vi "Teleop.vi"(10 "Match Info":T1={"Autonomous Elapsed Seconds"=0.0, "TeleOp Elapsed Seconds"=0.0, "Disabled Elapsed Seconds"=0.0, "Visited Autonomous"=FALSE, "Visited TeleOp"=FALSE, "Visited Disabled"=FALSE, "Autonomous Settings"={"Autonomous Style"=enum."Independent", "VI Refnum"=refnum}}, 11 "Call Context":T2) -> ()   [LabVIEW 2012]
doc: "This VI is called for each TeleOp packet received from the DS where the robot is not disabled. It is often used to read from the joysticks and update I/O or to update setpoints for timed control loops. It should complete and return within 20 milliseconds or it may miss DS packets."
uses:
  <vilib>/Rock Robotics/WPI/DriverStation/WPI_DriverStationDerivedRobotMode.ctl
  <vilib>/Rock Robotics/WPI/DriverStation/WPI_DriverStationMatch Info.ctl
  <vilib>/Rock Robotics/WPI/Relay/WPI_RelayValue.ctl
  Robot Global Data.vi
  <vilib>/Rock Robotics/WPI/Joystick/WPI_JoystickGetSetRefNum.vi
panel:
  in  "Numeric":dbl=0.87
  in  "Ext Const":dbl=0.5
  in  "Dep Const":dbl=1.0
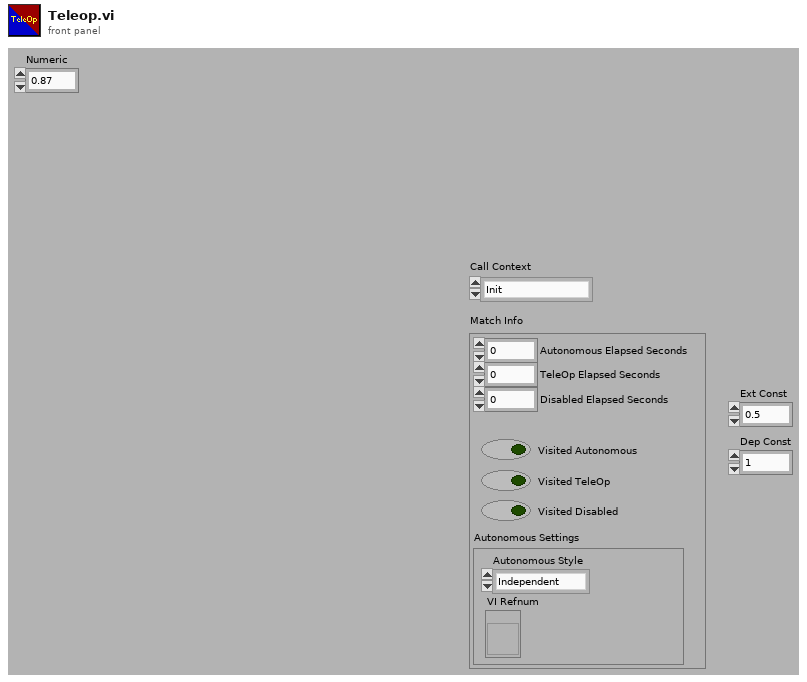
[diagram p1: front panel]
types:
  T1 = typedef "WPI_DriverStationMatch Info.ctl" = cluster{"Autonomous Elapsed Seconds":dbl, "TeleOp Elapsed Seconds":dbl, "Disabled Elapsed Seconds":dbl, "Visited Autonomous":bool, "Visited TeleOp":bool, "Visited Disabled":bool, "Autonomous Settings":cluster{"Autonomous Style":enum16{"Iterative", "Independent"}, "VI Refnum":refnum<vi>}}
  T2 = typedef "WPI_DriverStationDerivedRobotMode.ctl" = enum16{"Init", "Execute", "Stop"}
  T3 = typedef "WPI_RelayValue.ctl" = enum16{"Off", "On", "Forward", "Reverse"}
  T4 = cluster{"Driver Station Digital Input (1-8)[0]":bool, "Driver Station Digital Input (1-8)[1]":bool, "Driver Station Digital Input (1-8)[2]":bool, "Driver Station Digital Input (1-8)[3]":bool, "Driver Station Digital Input (1-8)[4]":bool, "Driver Station Digital Input (1-8)[5]":bool, "Driver Station Digital Input (1-8)[6]":bool, "Driver Station Digital Input (1-8)[7]":bool, "Driver Station Digital Input (1-8)[8]":bool}
  T5 = typedef "WPI_DigitalInputDevRef.ctl" = cluster{"DevStatus":errorcluster, "DIO Channel":T6, "Digital Module":T7}
  T6 = typedef "FPGA_DIOChannel.ctl" = enum8{"DIO 1", "DIO 2", "DIO 3", "DIO 4", "DIO 5", "DIO 6", "DIO 7", "DIO 8", "DIO 9", "DIO 10", "DIO 11", "DIO 12", "DIO 13", "DIO 14", "Invalid"}
  T7 = typedef "FPGA_TypedefDigitalModule.ctl" = enum16{"Digital Module 1", "Digital Module 2"}
  T8 = cluster{"Right Servo High":dbl, "Right Servo Mid":dbl, "Right Servo Low":dbl, "Left Servo High":dbl, "Left Servo Mid":dbl, "Left Servo Low":dbl}
  T9 = typedef "WPI_JoystickDevRef.ctl" = cluster{"Device":T10}
  T10 = typedef "WPI_JoystickDeviceEnum.ctl" = enum16{"USB 1", "USB 2", "USB 3", "USB 4", "Kinect 1", "Kinect 2"}
  T11 = cluster{"axis 1 (x)":dbl, "axis 2 (y)":dbl, "axis 3 (throttle)":dbl, "axis 4":dbl, "axis 5":dbl, "axis 6":dbl}
  T12 = typedef "WPI_RelayDevRef.ctl" = cluster{"DevStatus":errorcluster, "Relay Channel":T13, "Digital Module":T7, "Relay Direction":T14}
  T13 = typedef "FPGA_DIORelayChannel.ctl" = enum8{"Relay 1", "Relay 2", "Relay 3", "Relay 4", "Relay 5", "Relay 6", "Relay 7", "Relay 8", "Invalid"}
  T14 = typedef "WPI_RelayDirection.ctl" = enum16{"Both directions", "Forward only", "Reverse only"}
  T15 = typedef "WPI_ServoDeviceRef.ctl" = cluster{"DeviceStatus":errorcluster, "Digital Module":T7, "PWM Channel":T16, "DeadBand":T17}
  T16 = typedef "FPGA_DIOPWMChannel.ctl" = enum8{"PWM 1", "PWM 2", "PWM 3", "PWM 4", "PWM 5", "PWM 6", "PWM 7", "PWM 8", "PWM 9", "PWM 10", "Invalid"}
  T17 = typedef "WPI_PWMDeadband.ctl" = cluster{"Name":string, "maxPositivePwm":i32, "minPositivePwm":i32, "centerPwm":i32, "maxNegativePwm":i32, "minNegativePwm":i32, "angularRange":u16}
  T18 = typedef "WPI_MotorControlDeviceRef.ctl" = cluster{"DeviceStatus":errorcluster, "Type":enum16{"PWM", "CAN"}, "PWM":cluster{"Digital Module":T7, "PWM Channel":T16, "DeadBand":T17}, "CAN":cluster{"Device Number":u8, "Control Mode":T19, "Semaphore":T20, "Max Vout":dbl}, "Invert":bool, "TransformRef":T21, "InvTransformRef":T21}
  T19 = typedef "WPI_CANJaguar_ControlMode.ctl" = enum8{"Percent VBus", "Current", "Speed", "Position", "Voltage"}
  T20 = typedef "Semaphore RefNum" = refnum<k1>
  T21 = typedef "WPI_PWMTransform_ConPane.ctl" = refnum<vi>
  T22 = typedef "WPI_JoystickButtonState.ctl" = cluster{"Button 1":bool, "Button 2":bool, "Button 3":bool, "Button 4":bool, "Button 5":bool, "Button 6":bool, "Button 7":bool, "Button 8":bool, "Button 9":bool, "Button 10":bool, "Button 11":bool, "Button 12":bool}
  T23 = cluster{"FlipperLeftUp":dbl, "FlipperLeftDown":dbl, "FlipperRightUp":dbl, "FlipperRightDown":dbl, "KickerLeftBack":dbl, "KickerLeftForward":dbl, "KickerRightBack":dbl, "KickerRightForward":dbl}
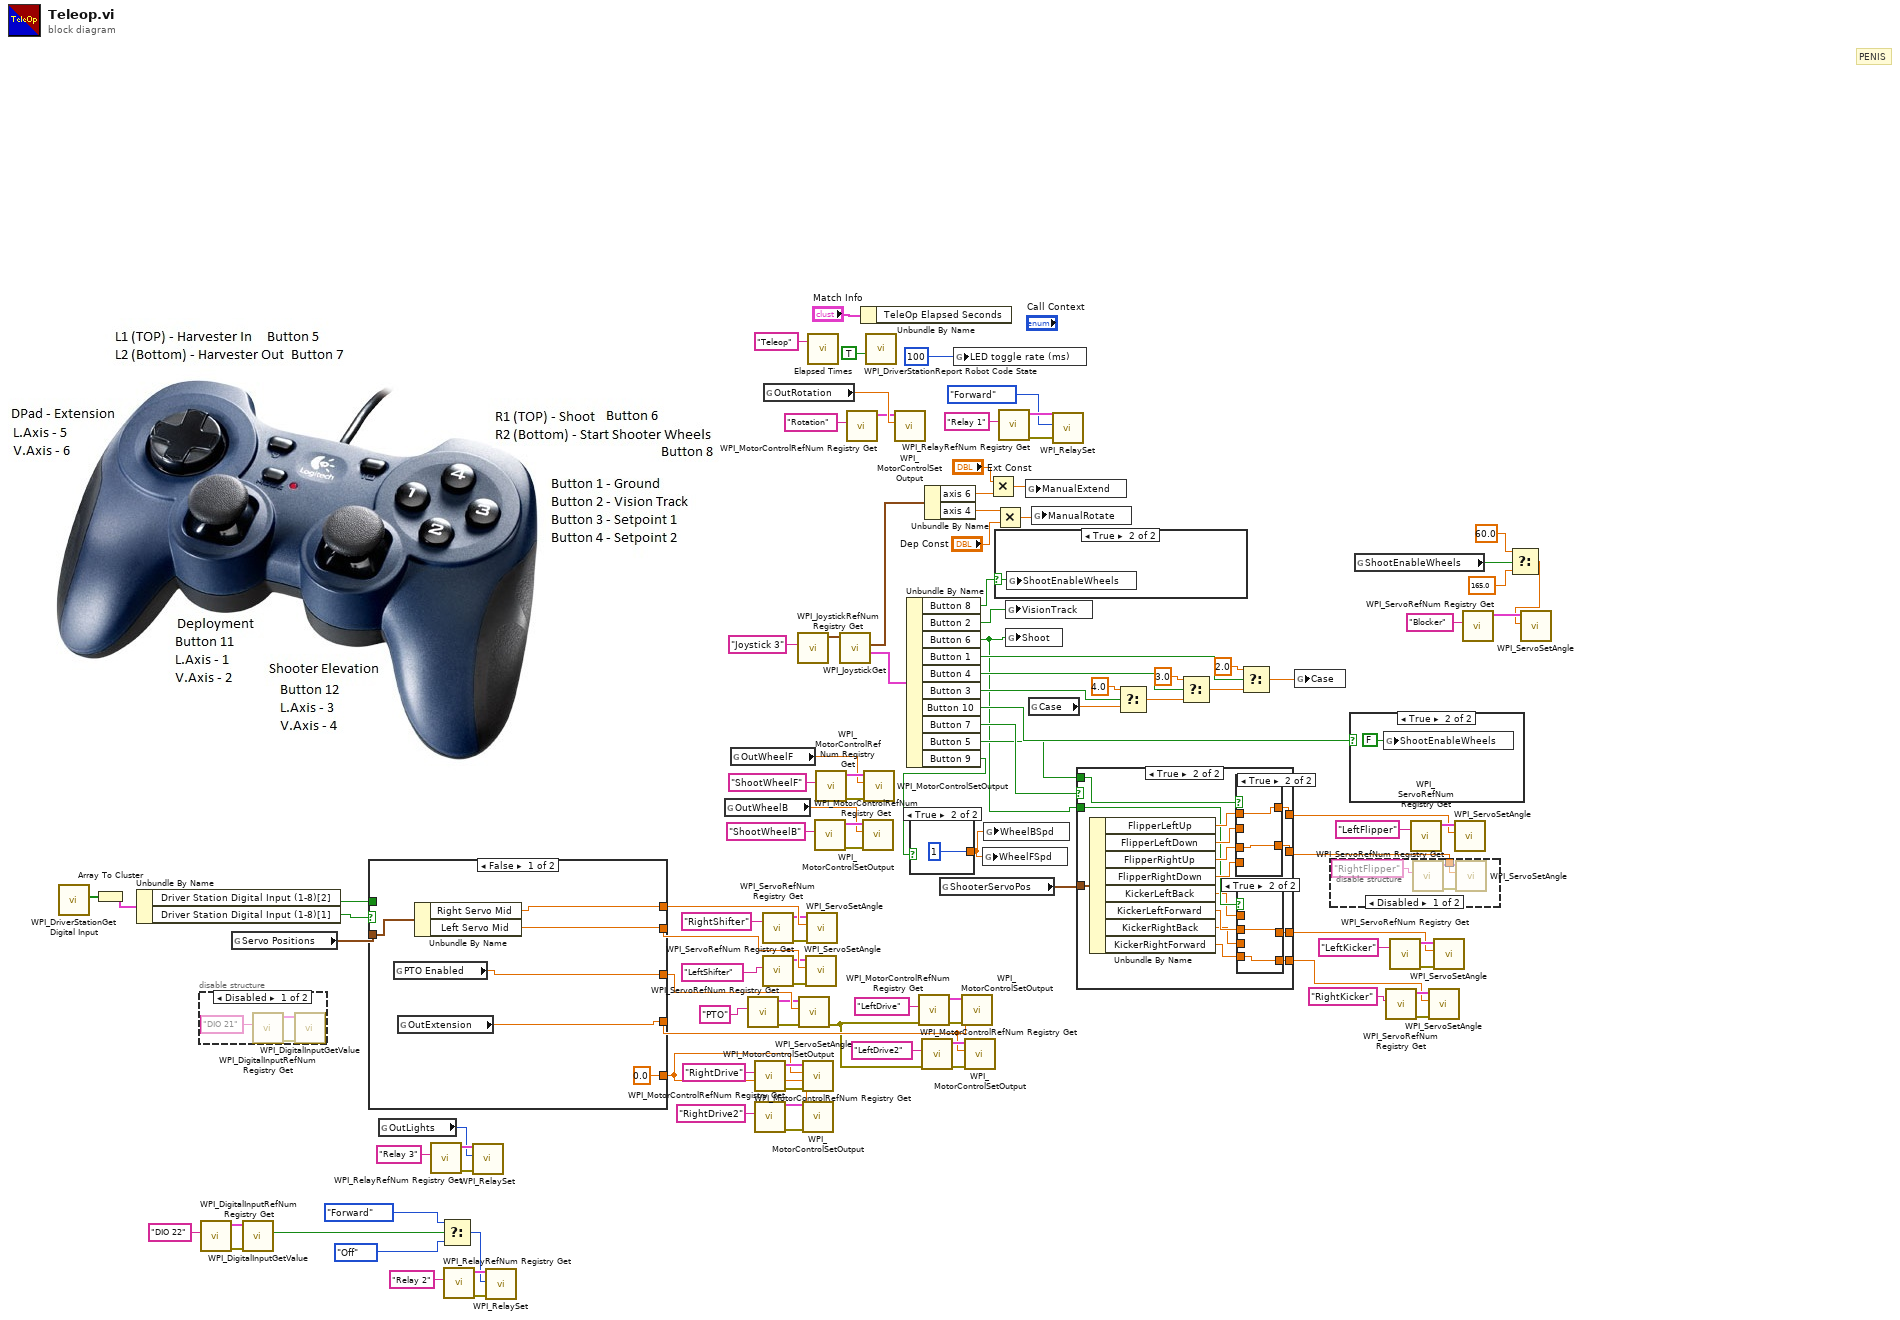
[diagram p0: block diagram]
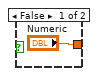
[diagram p3: hidden frame]
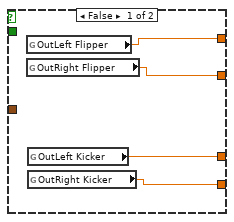
[diagram p5: hidden frame]
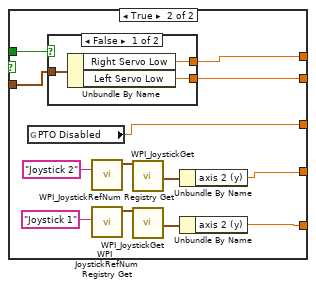
[diagram p8: hidden frame]
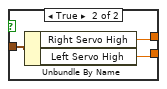
[diagram p9: hidden frame]
diagram:
  # "PENIS"
  n1 = call <vilib>:"WPI_DriverStationGet Digital Input.vi"() -> ("Driver Station Digital Input (1-8)"=w80:bool[])  [unwired: 11 in]
  n2 = Array To Cluster(array=w80) -> (cluster=w79:T4)
  n3 = Unbundle By Name(w79) -> ("Driver Station Digital Input (1-8)[2]"=w78:bool, "Driver Station Digital Input (1-8)[1]"=w18:bool)
  n4 = disable-structure shown="Disabled" {
    frame Disabled {
      n5 = call <vilib>:"WPI_DigitalInputRefNum Registry Get.vi"("refnum name"="DIO 21") -> ("error out"=w113:errorcluster, "DigitalInputDevRef"=w114:T5)  [unwired: 9 in]
      n6 = call <vilib>:"WPI_DigitalInputGetValue.vi"("error in (no error)"=w113, "DigitalInputDevRef"=w114) -> ()  [unwired: 7 in, 3 out]
    }
    frame Enabled {
    }
  }
  n7 = call <vilib>:"WPI_DigitalInputRefNum Registry Get.vi"("refnum name"="DIO 22") -> ("error out"=w12:errorcluster, "DigitalInputDevRef"=w8:T5)  [unwired: 9 in]
  n8 = global read "Robot Global Data.vi" "Servo Positions"() -> (w77:T8)
  n9 = call <vilib>:"WPI_DigitalInputGetValue.vi"("error in (no error)"=w12, "DigitalInputDevRef"=w8) -> ("Value"=w11:bool)  [unwired: 7 in, 2 out]
  n10 = case shown="False" w18 {
    tunnel: w78 -> [_ w134]
    tunnel: w77 -> [w121 w133]
    tunnel: [w120 w132] -> w76
    tunnel: [w119 w131] -> w75
    tunnel: [w118 w130] -> w68
    tunnel: [w116 w123] -> w67
    tunnel: [0.0 w122] -> w66
    frame False {
      n11 = global read "Robot Global Data.vi" "PTO Enabled"() -> (w118:dbl)
      n12 = global read "Robot Global Data.vi" "OutExtension"() -> (w116:dbl)
      n13 = Unbundle By Name(w121) -> ("Right Servo Mid"=w120:dbl, "Left Servo Mid"=w119:dbl)
    }
    frame True {
      n14 = global read "Robot Global Data.vi" "PTO Disabled"() -> (w130:dbl)
      n15 = case shown="False" w134 {
        tunnel: w133 -> [w137 w140]
        tunnel: [w136 w139] -> w132
        tunnel: [w135 w138] -> w131
        frame False {
          n16 = Unbundle By Name(w137) -> ("Right Servo Low"=w136:dbl, "Left Servo Low"=w135:dbl)
        }
        frame True {
          n17 = Unbundle By Name(w140) -> ("Right Servo High"=w139:dbl, "Left Servo High"=w138:dbl)
        }
      }
      n18 = call <vilib>:"WPI_JoystickRefNum Registry Get.vi"("refnum name"="Joystick 2") -> ("JoystickDevRef"=w124:T9)  [unwired: 1 in, 9 out]
      n19 = call <vilib>:"WPI_JoystickRefNum Registry Get.vi"("refnum name"="Joystick 1") -> ("JoystickDevRef"=w128:T9)  [unwired: 1 in, 9 out]
      n20 = call <vilib>:"WPI_JoystickGet.vi"("JoystickDevRef"=w124) -> ("Axes"=w126:T11)  [unwired: 1 in, 5 out]
      n21 = call <vilib>:"WPI_JoystickGet.vi"("JoystickDevRef"=w128) -> ("Axes"=w129:T11)  [unwired: 1 in, 5 out]
      n22 = Unbundle By Name(w126) -> ("axis 2 (y)"=w123:dbl)
      n23 = Unbundle By Name(w129) -> ("axis 2 (y)"=w122:dbl)
    }
  }
  n24 = global read "Robot Global Data.vi" "OutLights"() -> (w17:T3)
  n25 = call <vilib>:"WPI_RelayRefNum Registry Get.vi"("refnum name"="Relay 3") -> ("error out"=w51:errorcluster, "RelayDevRef"=w49:T12)  [unwired: 9 in]
  n26 = Select(t=WPI_RelayValue."Forward" ("RelayValue"), s=w11, f=WPI_RelayValue."Off" ("RelayValue")) -> (s? t:f=w7:T3)
  n27 = call <vilib>:"WPI_RelayRefNum Registry Get.vi"("refnum name"="Relay 2") -> ("error out"=w14:errorcluster, "RelayDevRef"=w16:T12)  [unwired: 9 in]
  n28 = call <vilib>:"WPI_RelaySet.vi"("error in (no error)"=w51, "RelayValue"=w17, "RelayDevRef"=w49) -> ()  [unwired: 7 in, 2 out]
  n29 = call <vilib>:"WPI_RelaySet.vi"("error in (no error)"=w14, "RelayValue"=w7, "RelayDevRef"=w16) -> ()  [unwired: 7 in, 2 out]
  n30 = global read "Robot Global Data.vi" "OutWheelB"() -> (w38:dbl)
  n31 = global read "Robot Global Data.vi" "OutWheelF"() -> (w39:dbl)
  n32 = call <vilib>:"WPI_ServoRefNum Registry Get.vi"("refnum name"="PTO") -> ("error out"=w61:errorcluster, "ServoDeviceRef"=w62:T15)  [unwired: 9 in]
  n33 = call <vilib>:"WPI_MotorControlRefNum Registry Get.vi"("refnum name"="RightDrive") -> ("error out"=w90:errorcluster, "MotorControlDevRef"=w92:T18)  [unwired: 9 in]
  n34 = call <vilib>:"WPI_MotorControlRefNum Registry Get.vi"("refnum name"="RightDrive2") -> ("error out"=w83:errorcluster, "MotorControlDevRef"=w81:T18)  [unwired: 9 in]
  n35 = call <vilib>:"WPI_ServoRefNum Registry Get.vi"("refnum name"="RightShifter") -> ("error out"=w71:errorcluster, "ServoDeviceRef"=w72:T15)  [unwired: 9 in]
  n36 = call <vilib>:"WPI_ServoRefNum Registry Get.vi"("refnum name"="LeftShifter") -> ("error out"=w73:errorcluster, "ServoDeviceRef"=w74:T15)  [unwired: 9 in]
  n37 = global read "Robot Global Data.vi" "OutRotation"() -> (w65:dbl)
  n38 = call <vilib>:"WPI_JoystickRefNum Registry Get.vi"("refnum name"="Joystick 3") -> ("JoystickDevRef"=w109:T9)  [unwired: 9 in, 1 out]
  n39 = call <vilib>:"WPI_ServoSetAngle.vi"("error in (no error)"=w61, "Angle"=w68, "ServoDeviceRef"=w62) -> ("error out"=w57:errorcluster)  [unwired: 7 in, 1 out]
  n40 = call <vilib>:"WPI_MotorControlSetOutput.vi"("error in (no error)"=w90, "Output"=w66, "MotorControlDevRef"=w92) -> ()  [unwired: 6 in, 3 out]
  n41 = call <vilib>:"WPI_MotorControlSetOutput.vi"("error in (no error)"=w83, "Output"=w66, "MotorControlDevRef"=w81) -> ()  [unwired: 6 in, 3 out]
  n42 = call <vilib>:"WPI_ServoSetAngle.vi"("error in (no error)"=w73, "Angle"=w75, "ServoDeviceRef"=w74) -> ()  [unwired: 7 in, 2 out]
  n43 = call <vilib>:"WPI_ServoSetAngle.vi"("error in (no error)"=w71, "Angle"=w76, "ServoDeviceRef"=w72) -> ()  [unwired: 7 in, 2 out]
  n44 = call "Elapsed Times.vi"("Call Name"="Teleop") -> ()  [unwired: 2 in, 1 out]
  n45 = call <vilib>:"WPI_MotorControlRefNum Registry Get.vi"("refnum name"="ShootWheelB") -> ("error out"=w41:errorcluster, "MotorControlDevRef"=w42:T18)  [unwired: 9 in]
  n46 = call <vilib>:"WPI_MotorControlRefNum Registry Get.vi"("refnum name"="ShootWheelF") -> ("error out"=w43:errorcluster, "MotorControlDevRef"=w40:T18)  [unwired: 9 in]
  n47 = call <vilib>:"WPI_JoystickGet.vi"("JoystickDevRef"=w109) -> ("Buttons"=w107:T22, "Axes"=w106:T11)  [unwired: 4 in, 1 out]
  n48 = call <vilib>:"WPI_MotorControlRefNum Registry Get.vi"("refnum name"="Rotation") -> ("MotorControlDevRef"=w63:T18)  [unwired: 9 in, 1 out]
  n49 = Unbundle By Name("Match Info") -> ()  [unwired: 1 out]
  n50 = call <vilib>:"WPI_MotorControlSetOutput.vi"("error in (no error)"=w41, "Output"=w38, "MotorControlDevRef"=w42) -> ()  [unwired: 6 in, 3 out]
  n51 = call <vilib>:"WPI_MotorControlSetOutput.vi"("error in (no error)"=w43, "Output"=w39, "MotorControlDevRef"=w40) -> ()  [unwired: 6 in, 3 out]
  n52 = call <vilib>:"WPI_DriverStationReport Robot Code State.vi"("TeleOp"=TRUE ("Autonomous")) -> ()  [unwired: 10 in, 1 out]
  n53 = call <vilib>:"WPI_MotorControlSetOutput.vi"("Output"=w65, "MotorControlDevRef"=w63) -> ()  [unwired: 7 in, 3 out]
  n54 = Unbundle By Name(w107) -> ("Button 8"=w94:bool, "Button 2"=w105:bool, "Button 6"=w22:bool, "Button 1"=w104:bool, "Button 4"=w102:bool, "Button 3"=w101:bool, "Button 10"=w37:bool, "Button 7"=w36:bool, "Button 5"=w35:bool, "Button 9"=w19:bool)
  n55 = case shown="True" w19 {
    tunnel: ["Numeric" 1] -> w20
    frame False {
    }
    frame True {
    }
  }
  n56 = call <vilib>:"WPI_MotorControlRefNum Registry Get.vi"("error in (no error)"=w57, "refnum name"="LeftDrive") -> ("error out"=w85:errorcluster, "MotorControlDevRef"=w88:T18)  [unwired: 8 in]
  n57 = call <vilib>:"WPI_MotorControlRefNum Registry Get.vi"("error in (no error)"=w57, "refnum name"="LeftDrive2") -> ("error out"=w84:errorcluster, "MotorControlDevRef"=w86:T18)  [unwired: 8 in]
  n58 = Unbundle By Name(w106) -> ("axis 6"=w48:dbl, "axis 4"=w58:dbl)
  n59 = global read "Robot Global Data.vi" "ShooterServoPos"() -> (w23:T23)
  n60 = global write "Robot Global Data.vi" "LED toggle rate (ms)"(u32 100 ("LED ms toggle rate")) -> ()
  n61 = call <vilib>:"WPI_MotorControlSetOutput.vi"("error in (no error)"=w85, "Output"=w67, "MotorControlDevRef"=w88) -> ()  [unwired: 6 in, 3 out]
  n62 = call <vilib>:"WPI_MotorControlSetOutput.vi"("error in (no error)"=w84, "Output"=w67, "MotorControlDevRef"=w86) -> ()  [unwired: 6 in, 3 out]
  n63 = global write "Robot Global Data.vi" "WheelFSpd"(w20) -> ()
  n64 = global write "Robot Global Data.vi" "WheelBSpd"(w20) -> ()
  n65 = Multiply(x="Ext Const", y=w48) -> (x*y=w46:dbl)
  n66 = Multiply(x=w58, y="Dep Const") -> (x*y=w56:dbl)
  n67 = case shown="True" w94 {
    selector: w94 -> [_ w143]
    frame False {
    }
    frame True {
      n68 = global write "Robot Global Data.vi" "ShootEnableWheels"(w143) -> ()
    }
  }
  n69 = call <vilib>:"WPI_RelayRefNum Registry Get.vi"("refnum name"="Relay 1") -> ("error out"=w53:errorcluster, "RelayDevRef"=w55:T12)  [unwired: 9 in]
  n70 = global write "Robot Global Data.vi" "VisionTrack"(w105) -> ()
  n71 = global write "Robot Global Data.vi" "Shoot"(w22) -> ()
  n72 = global write "Robot Global Data.vi" "ManualExtend"(w46) -> ()
  n73 = global read "Robot Global Data.vi" "Case"() -> (w96:dbl)
  n74 = global write "Robot Global Data.vi" "ManualRotate"(w56) -> ()
  n75 = call <vilib>:"WPI_RelaySet.vi"("error in (no error)"=w53, "RelayValue"=WPI_RelayValue."Forward", "RelayDevRef"=w55) -> ()  [unwired: 7 in, 2 out]
  n76 = case shown="True" w36 {
    tunnel: w35 -> [_ w148]
    tunnel: [w147 w161] -> w26
    tunnel: [w146 w159] -> w25
    tunnel: [w145 w150] -> w24
    tunnel: [w144 w149] -> w21
    tunnel: w23 -> [_ w162]
    tunnel: w22 -> [_ w155]
    frame False {
      n77 = global read "Robot Global Data.vi" "OutLeft Flipper"() -> (w147:dbl)
      n78 = global read "Robot Global Data.vi" "OutRight Flipper"() -> (w146:dbl)
      n79 = global read "Robot Global Data.vi" "OutLeft Kicker"() -> (w145:dbl)
      n80 = global read "Robot Global Data.vi" "OutRight Kicker"() -> (w144:dbl)
    }
    frame True {
      n81 = Unbundle By Name(w162) -> ("FlipperLeftUp"=w160:dbl, "FlipperLeftDown"=w157:dbl, "FlipperRightUp"=w158:dbl, "FlipperRightDown"=w156:dbl, "KickerLeftBack"=w154:dbl, "KickerLeftForward"=w153:dbl, "KickerRightBack"=w152:dbl, "KickerRightForward"=w151:dbl)
      n82 = case shown="True" w148 {
        tunnel: [w168 w170] -> w161
        tunnel: w160 -> [_ w170]
        tunnel: [w167 w169] -> w159
        tunnel: w158 -> [_ w169]
        tunnel: w157 -> [w168 _]
        tunnel: w156 -> [w167 _]
        frame False {
        }
        frame True {
        }
      }
      n83 = case shown="True" w155 {
        tunnel: w154 -> [w164 _]
        tunnel: w153 -> [_ w165]
        tunnel: w152 -> [w163 _]
        tunnel: w151 -> [_ w166]
        tunnel: [w164 w165] -> w150
        tunnel: [w163 w166] -> w149
        frame False {
        }
        frame True {
        }
      }
    }
  }
  n84 = Select(t=4.0, s=w101, f=w96) -> (s? t:f=w100:dbl)
  n85 = Select(t=3.0, s=w102, f=w100) -> (s? t:f=w98:dbl)
  n86 = Select(t=2.0, s=w104, f=w98) -> (s? t:f=w95:dbl)
  n87 = global write "Robot Global Data.vi" "Case"(w95) -> ()
  n88 = disable-structure shown="Disabled" {
    disable-tunnel: w25 -> [w171 _]
    frame Disabled {
      n89 = call <vilib>:"WPI_ServoRefNum Registry Get.vi"("refnum name"="RightFlipper") -> ("error out"=w174:errorcluster, "ServoDeviceRef"=w172:T15)  [unwired: 9 in]
      n90 = call <vilib>:"WPI_ServoSetAngle.vi"("error in (no error)"=w174, "Angle"=w171, "ServoDeviceRef"=w172) -> ()  [unwired: 7 in, 2 out]
    }
    frame Enabled {
    }
  }
  n91 = case shown="True" w37 {
    frame False {
    }
    frame True {
      n92 = global write "Robot Global Data.vi" "ShootEnableWheels"(FALSE ("ShootStartWheels")) -> ()
    }
  }
  n93 = global read "Robot Global Data.vi" "ShootEnableWheels"() -> (w4:bool)
  n94 = call <vilib>:"WPI_ServoRefNum Registry Get.vi"("refnum name"="RightKicker") -> ("error out"=w33:errorcluster, "ServoDeviceRef"=w31:T15)  [unwired: 9 in]
  n95 = call <vilib>:"WPI_ServoRefNum Registry Get.vi"("refnum name"="LeftKicker") -> ("error out"=w27:errorcluster, "ServoDeviceRef"=w28:T15)  [unwired: 9 in]
  n96 = call <vilib>:"WPI_ServoRefNum Registry Get.vi"("refnum name"="LeftFlipper") -> ("ServoDeviceRef"=w29:T15)  [unwired: 9 in, 1 out]
  n97 = call <vilib>:"WPI_ServoSetAngle.vi"("error in (no error)"=w33, "Angle"=w21, "ServoDeviceRef"=w31) -> ()  [unwired: 7 in, 2 out]
  n98 = call <vilib>:"WPI_ServoSetAngle.vi"("error in (no error)"=w27, "Angle"=w24, "ServoDeviceRef"=w28) -> ()  [unwired: 7 in, 2 out]
  n99 = call <vilib>:"WPI_ServoSetAngle.vi"("Angle"=w26, "ServoDeviceRef"=w29) -> ()  [unwired: 8 in, 2 out]
  n100 = call <vilib>:"WPI_ServoRefNum Registry Get.vi"("refnum name"="Blocker") -> ("ServoDeviceRef"=w5:T15)  [unwired: 9 in, 1 out]
  n101 = Select(t=60.0 ("f"), s=w4, f=165.0 ("t")) -> (s? t:f=w3:dbl)
  n102 = call <vilib>:"WPI_ServoSetAngle.vi"("Angle"=w3, "ServoDeviceRef"=w5) -> ()  [unwired: 8 in, 2 out]
